vi "labview_2_unix_conversion.vi"() -> ()   [LabVIEW 2018]
panel:
  out "lv_timestamp":dbl format="%.6f"
  out "lv_time_utc":timestamp
  out "lv_time_local":timestamp
  out "utc_timestamp":timestamp format="%^<%.3X\n%x>T"
  out "local_timstamp":timestamp
  in  "conversion_constant":i32
  out "unix_timestamp":dbl format="%.6f"
  out "lv2unix_conv_timestamp":dbl format="%.6f"
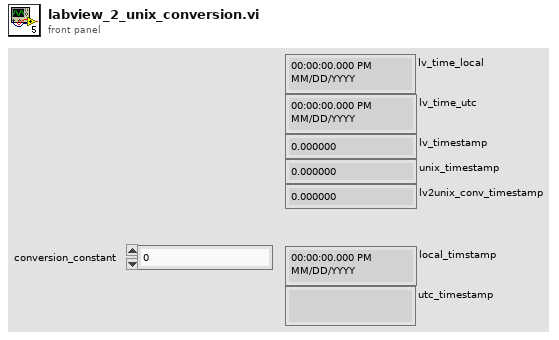
[diagram p1: front panel]
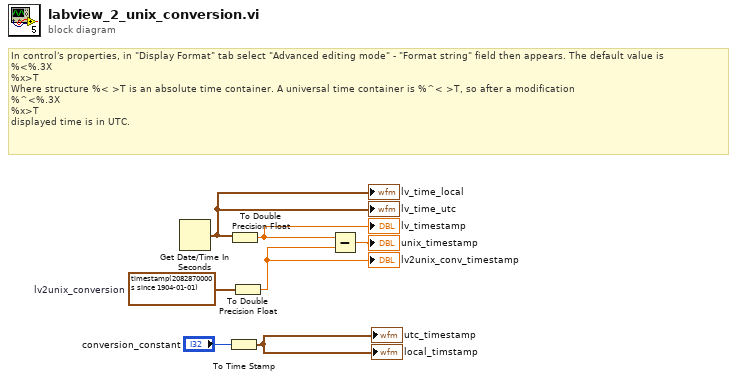
[diagram p0: block diagram]
diagram:
  w7 = timestamp(2082870000 s since 1904-01-01)  # lv2unix_conversion
  # "In control's properties, in \"Display Format\" tab select \"Advanced editing mode\" - \"Format string\" field then appears. The default value is \n%<%.3X\n%x>T\nWhere structure %< >T is an absolute time container. A universal time container is %^< >T, so after a modification\n%^<%.3X\n%x>T\ndisplayed time is in UTC."
  n1 = Get Date/Time In Seconds() -> (seconds since 1Jan1904=w1:timestamp)
  "lv_time_local" <- w1
  "lv_time_utc" <- w1
  n2 = To Time Stamp(1:"conversion_constant") -> (0:→"local_timstamp" →"utc_timestamp":timestamp)
  n3 = To Double Precision Float(number=w1) -> (double precision float=w2:dbl)
  "lv_timestamp" <- w2
  n4 = To Double Precision Float(number=w7) -> (double precision float=w6:dbl)
  "lv2unix_conv_timestamp" <- w6
  n5 = Subtract(x=w2, y=w6) -> (x-y=→"unix_timestamp":dbl)
